vi "Main.vi"() -> ()   [LabVIEW 2019]
doc: "The myRIO Project template acquires acceleration data from the onboard accelerometer and displays the changes of acceleration values in a waveform chart."
uses:
  <vilib>/myRIO/Instrument Drivers/Onboard IO/DIO/typedefs/DIO Reference.ctl
  <vilib>/myRIO/Common/Instrument Driver Framework/Utilities/typedefs/myRIO Generic Hardware Reference.ctl
  <vilib>/myRIO/Common/Instrument Driver Framework/Utilities/typedefs/Hardware Version Enum.ctl
  <vilib>/myRIO/Common/Instrument Driver Framework/Utilities/typedefs/myRIO v1.0 Reference.ctl
  <vilib>/myRIO/Common/Instrument Driver Framework/Utilities/typedefs/Generic FPGA Reference.ctl
  <vilib>/myRIO/Common/Instrument Driver Framework/myRIO v1.0/DIO/typedefs/DIO Channels List.ctl
  <vilib>/myRIO/Common/Instrument Driver Framework/myRIO v1.0/DIO/typedefs/DIO Channels Enum.ctl
  <vilib>/userDefined/High Color/nirio_resource_hc.ctl
  <vilib>/myRIO/Instrument Drivers/Onboard IO/AI/typedefs/AI Reference.ctl
  <vilib>/myRIO/Common/Instrument Driver Framework/myRIO v1.0/AI/typedefs/AI Channels List.ctl
  <vilib>/myRIO/Common/Instrument Driver Framework/myRIO v1.0/AI/typedefs/AI Channels Enum.ctl
  <vilib>/myRIO/Common/Instrument Driver Framework/Utilities/typedefs/Analog Scaling Constants List.ctl
  <vilib>/myRIO/Common/Instrument Driver Framework/Utilities/typedefs/Analog Scaling Constants.ctl
  <vilib>/myRIO/Common/Instrument Driver Framework/Utilities/vis/Is FPGA Ref Available.vi
  <vilib>/myRIO/Common/Instrument Driver Framework/myRIO v1.0/DIO/vis/myRIO v1.1 Open DIO.vi
  <vilib>/myRIO/Instrument Drivers/Onboard IO/DIO/vis/Write.vi
  <vilib>/myRIO/Instrument Drivers/Onboard IO/DIO/vis/Read.vi
  <vilib>/myRIO/Common/Instrument Driver Framework/myRIO v1.0/AI/vis/myRIO v1.1 Open AI.vi
  <vilib>/myRIO/Instrument Drivers/Onboard IO/AI/vis/Read.vi
  <vilib>/myRIO/Common/Instrument Driver Framework/Utilities/vis/Validate Channels.vi
  <vilib>/myRIO/Common/Instrument Driver Framework/myRIO v1.0/DIO/vis/myRIO v1.0 Reserve DIO.vi
  <vilib>/myRIO/Common/Instrument Driver Framework/myRIO v1.0/AI/vis/myRIO v1.0 Reserve AI.vi
  <vilib>/myRIO/Common/Instrument Driver Framework/myRIO v1.0/UART/vis/myRIO v1.0 Close UART.vi
  <vilib>/myRIO/Common/Instrument Driver Framework/myRIO v1.0/Resource Manager/vis/myRIO v1.0 Reserve Channel List.vi
  <vilib>/myRIO/Common/Instrument Driver Framework/myRIO v1.0/DIO/vis/myRIO v1.0 Build MUX Configuration DIO.vi
  <vilib>/myRIO/Common/Instrument Driver Framework/myRIO v1.0/AI/vis/myRIO v1.0 Build MUX Configuration AI.vi
  <vilib>/myRIO/Common/Instrument Driver Framework/myRIO v1.0/Resource Manager/vis/myRIO v1.0 Reserve Channel.vi
  <vilib>/myRIO/Common/Instrument Driver Framework/myRIO v1.0/Resource Manager/vis/myRIO v1.0 Unreserve Channel.vi
  <vilib>/myRIO/Common/Instrument Driver Framework/myRIO v1.0/Resource Manager/vis/myRIO v1.0 Create Configuration List.vi
  <vilib>/myRIO/Common/Instrument Driver Framework/myRIO v1.0/Resource Manager/vis/myRIO v1.0 Build Mutex Name.vi
  <vilib>/Utility/VariantDataType/GetNumericInfo.vi
  <vilib>/Utility/error.llb/Error Cluster From Error Code.vi
  <vilib>/myRIO/Common/Instrument Driver Framework/myRIO v1.0/myRIO v1.1 Open.vi
  <vilib>/myRIO/Common/Instrument Driver Framework/Utilities/vis/IO Manager.vi
  <vilib>/myRIO/Common/Instrument Driver Framework/Utilities/vis/Configuration Manager.vi
  <vilib>/myRIO/Common/Instrument Driver Framework/myRIO v1.0/Resource Manager/vis/myRIO v1.0 Configure IO.vi
  <vilib>/myRIO/Common/Instrument Driver Framework/myRIO v1.0/myRIO v1.0 Close.vi
  <vilib>/myRIO/Common/Instrument Driver Framework/myRIO v1.0/DIO/vis/myRIO v1.0 Write DIO.vi
  <vilib>/myRIO/Common/Instrument Driver Framework/myRIO v1.0/DIO/vis/myRIO v1.0 Read DIO.vi
  <vilib>/myRIO/Common/Instrument Driver Framework/myRIO v1.0/AI/vis/myRIO v1.0 Get Scaling Constants AI.vi
  <vilib>/myRIO/Common/Instrument Driver Framework/myRIO v1.0/AI/vis/myRIO v1.0 Read AI.vi
  <vilib>/myRIO/Common/Instrument Driver Framework/Utilities/vis/FPGA Ref Manager.vi
  <vilib>/myRIO/Common/Instrument Driver Framework/myRIO v1.0/myRIO v1.0 Reset FPGA.vi
  <vilib>/myRIO/Common/Instrument Driver Framework/myRIO v1.0/IRQ/vis/myRIO v1.0 IRQ Info FGV.vi
  <vilib>/myRIO/Common/Instrument Driver Framework/myRIO v1.0/IRQ/vis/myRIO v1.0 Timer IRQ Info FGV.vi
  <vilib>/myRIO/Common/Instrument Driver Framework/myRIO v1.0/IRQ/vis/myRIO v1.0 ISR Agent.vi
  <vilib>/myRIO/Instrument Drivers/Utilities/vis/Reset Index.vi
  <vilib>/myRIO/Common/Instrument Driver Framework/myRIO v1.0/Resource Manager/vis/myRIO v1.0 Block Write Resource Manager.vi
  <vilib>/myRIO/Express VI/Onboard IO/DO/DO Express VI.xnode
  <vilib>/myRIO/Instrument Drivers/Onboard IO/DIO/vis/myRIO DIO Open.xnode
  <vilib>/myRIO/Express VI/Onboard IO/DI/DI Express VI.xnode
  <vilib>/myRIO/Express VI/Onboard IO/AI/AI Express VI.xnode
  <vilib>/myRIO/Instrument Drivers/Onboard IO/AI/vis/myRIO AI Open.xnode
  <vilib>/myRIO/Instrument Drivers/Onboard IO/DIO/DIO.lvlib
  <vilib>/myRIO/Instrument Drivers/Onboard IO/AI/AI.lvlib
  <vilib>/myRIO/Instrument Drivers/Utilities/Utilities.lvlib
panel:
  out "Array - String":string[](array[string])
  out "Numeric":dbl
  in  "Go":bool
  in  "Single/Continuous":bool
  out "INPOS":bool
  in  "Home":bool
  in  "OFF/ON":bool
  in  "L/R":bool
  out "Index":i8=-1
  in  "Displacement (cm)":u8(slide) step=2 scale=0.0..10.0
  in  "Acceleration (m/s^2)":u8(slide)=1 min=1 max=5 step=1 scale=1.0..5.0
  out "Encoder Output (V)":dbl(graph)
  out "error out":errorcluster
  in  "Stop":bool
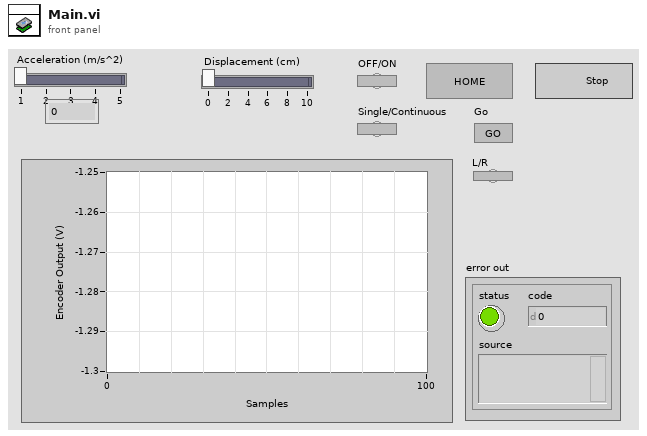
[diagram p1: front panel]
types:
  T1 = typedef "DIO.lvlib/DIO Reference.ctl" = cluster{"myRIO Reference":T2, "DIO Channels List":T6}
  T2 = typedef "myRIO Generic Hardware Reference.ctl" = cluster{"myRIO Model":T3, "myRIO Hardware Reference":T4}
  T3 = typedef "Hardware Version Enum.ctl" = enum16{"Unknown", "myRIO-1900", "myRIO-1950", "roboRIO", "NI ELVIS RIO CM", "ELVIS III"}
  T4 = typedef "myRIO v1.0 Reference.ctl" = cluster{"Generic FPGA Reference":T5, "Allow multiple opens":bool}
  T5 = typedef "Generic FPGA Reference.ctl" = refnum<k20>
  T6 = typedef "DIO Channels List.ctl" = T7[]
  T7 = typedef "DIO Channels Enum.ctl" = enum16{"Not Connected", "C/DIO0", "C/DIO1", "C/DIO2", "C/DIO3", "C/DIO4", "C/DIO5", "C/DIO6", "C/DIO7", "A/DIO0", "A/DIO1", "A/DIO2", "A/DIO3", "A/DIO4", "A/DIO5", "A/DIO6", "A/DIO7", "A/DIO8", "A/DIO9", "A/DIO10", "A/DIO11", "A/DIO12", "A/DIO13", "A/DIO14", "A/DIO15", "A/DIO16", "A/DIO17", "A/DIO18", "A/DIO19", "B/DIO0", "B/DIO1", "B/DIO2", "B/DIO3", "B/DIO4", "B/DIO5", "B/DIO6", "B/DIO7", "B/DIO8", "B/DIO9", "B/DIO10", "B/DIO11", "B/DIO12", "B/DIO13", "B/DIO14", "B/DIO15", "B/DIO16", "B/DIO17", "B/DIO18", "B/DIO19", "LED0", "LED1", "LED2", "LED3", "Button0", "DIO/DIO0", "DIO/DIO1", "DIO/DIO2", "DIO/DIO3", "DIO/DIO4", "DIO/DIO5", "DIO/DIO6", "DIO/DIO7", "DIO/DIO8", "DIO/DIO9", "SPI/CS0", "SPI/CS1", "SPI/CS2", "SPI/CS3", "LED RADIO (Green)", "LED RADIO (Red)", "LED COMM (Green)", "LED COMM (Red)", "LED MODE (Green)", "LED MODE (Red)"}
  T8 = typedef "nirio_resource_hc.ctl" = tag
  T9 = typedef "AI.lvlib/AI Reference.ctl" = cluster{"myRIO Reference":T2, "AI Channels List":T10, "AI Scaling Constants List":T12}
  T10 = typedef "AI Channels List.ctl" = T11[]
  T11 = typedef "AI Channels Enum.ctl" = enum16{"Not Connected", "AudioIn/Left", "AudioIn/Right", "C/AI0", "C/AI1", "A/AI0", "A/AI1", "A/AI2", "A/AI3", "A/AI4", "A/AI5", "A/AI6", "A/AI7", "B/AI0", "B/AI1", "B/AI2", "B/AI3", "B/AI4", "B/AI5", "B/AI6", "B/AI7", "AI/AI0", "AI/AI1", "AI/AI2", "AI/AI3", "A/AI0 (DIFF)", "A/AI1 (DIFF)", "A/AI2 (DIFF)", "A/AI3 (DIFF)", "B/AI0 (DIFF)", "B/AI1 (DIFF)", "B/AI2 (DIFF)", "B/AI3 (DIFF)"}
  T12 = typedef "Analog Scaling Constants List.ctl" = T13[]
  T13 = typedef "Analog Scaling Constants.ctl" = cluster{"LSB Weight (Volts)":dbl, "Offset (Volts)":dbl, "Signed?":bool}
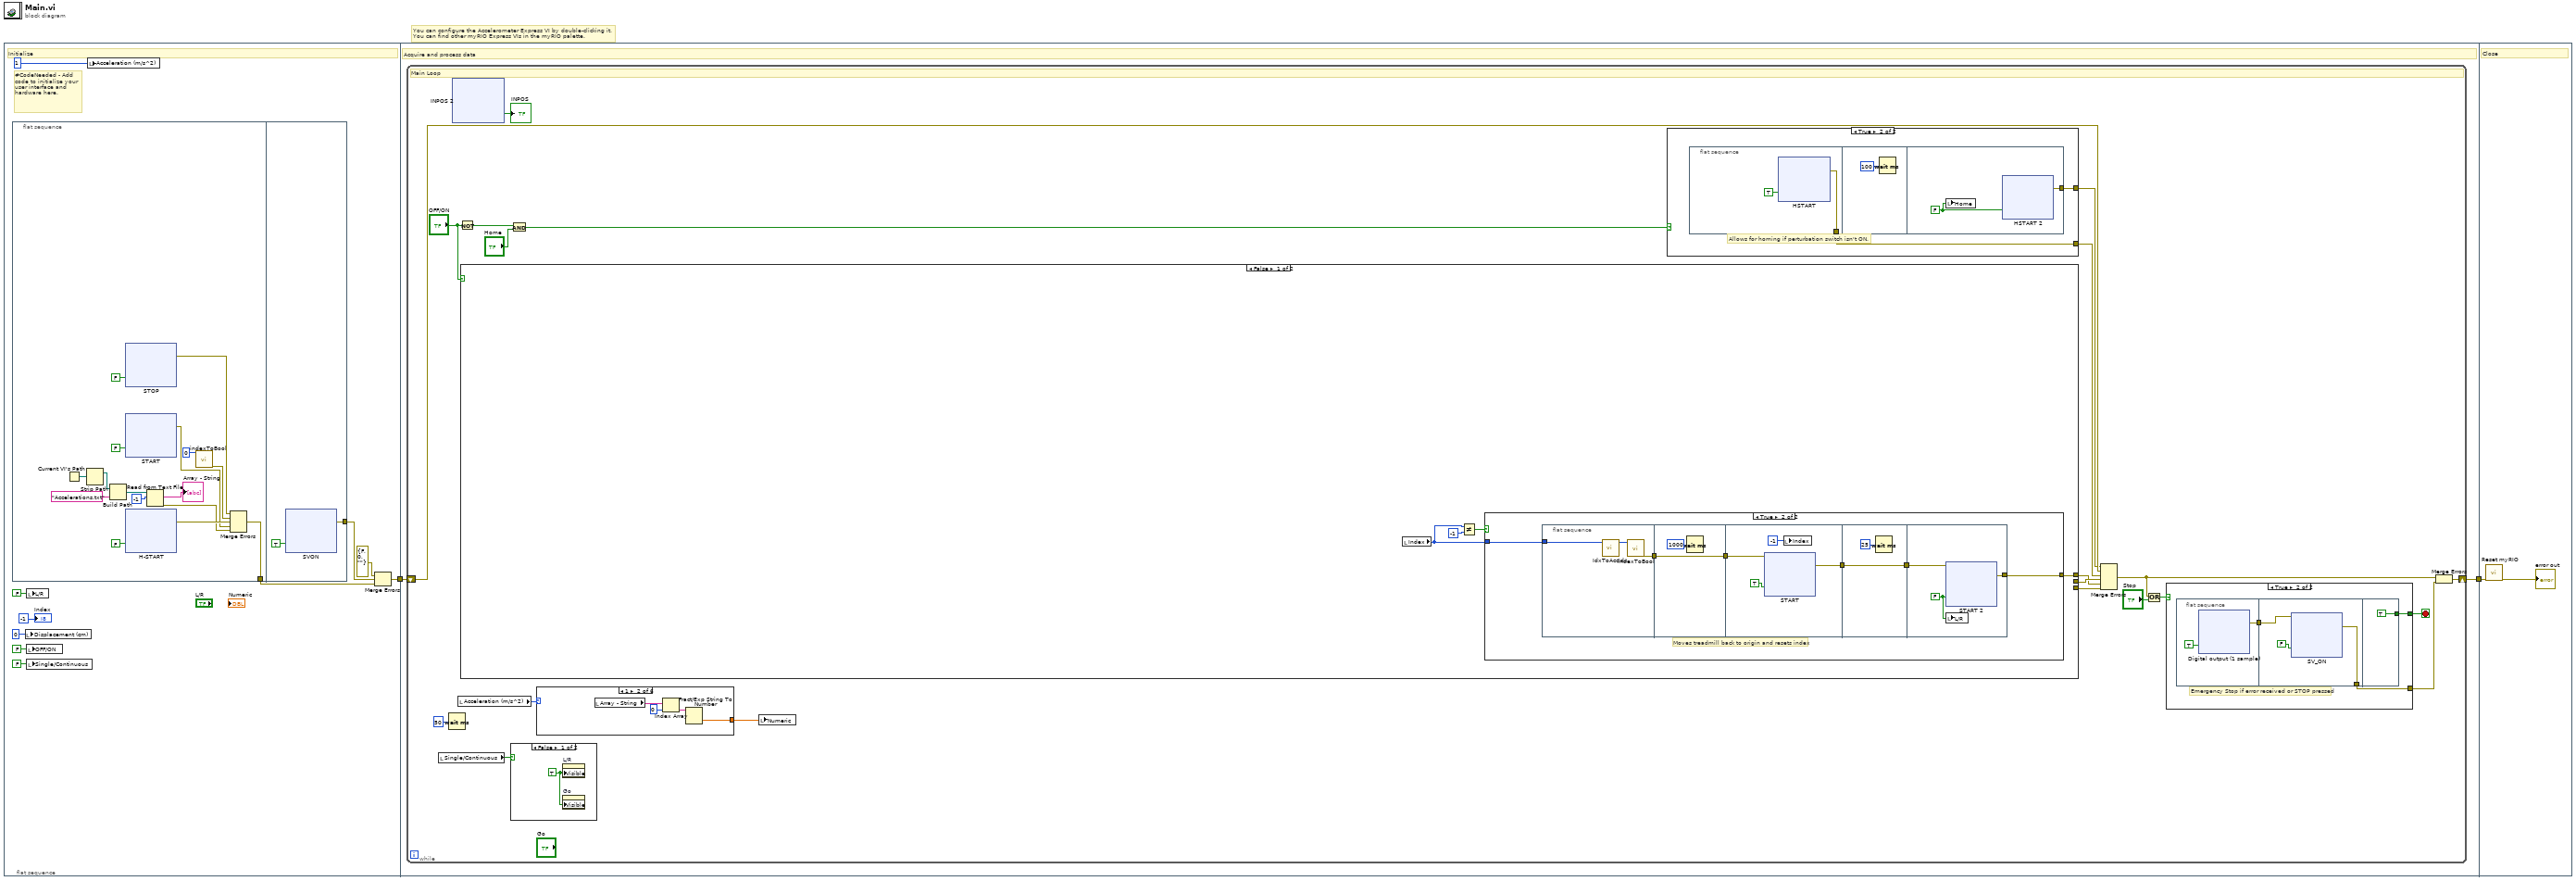
[diagram p0: block diagram]
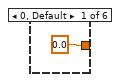
[diagram p2: hidden frame]
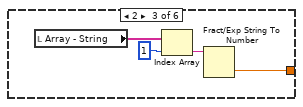
[diagram p3: hidden frame]
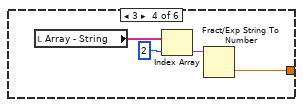
[diagram p4: hidden frame]
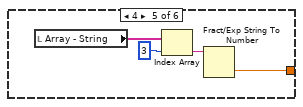
[diagram p5: hidden frame]
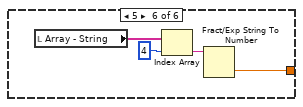
[diagram p6: hidden frame]
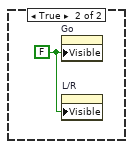
[diagram p7: hidden frame]
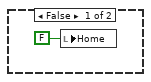
[diagram p9: hidden frame]
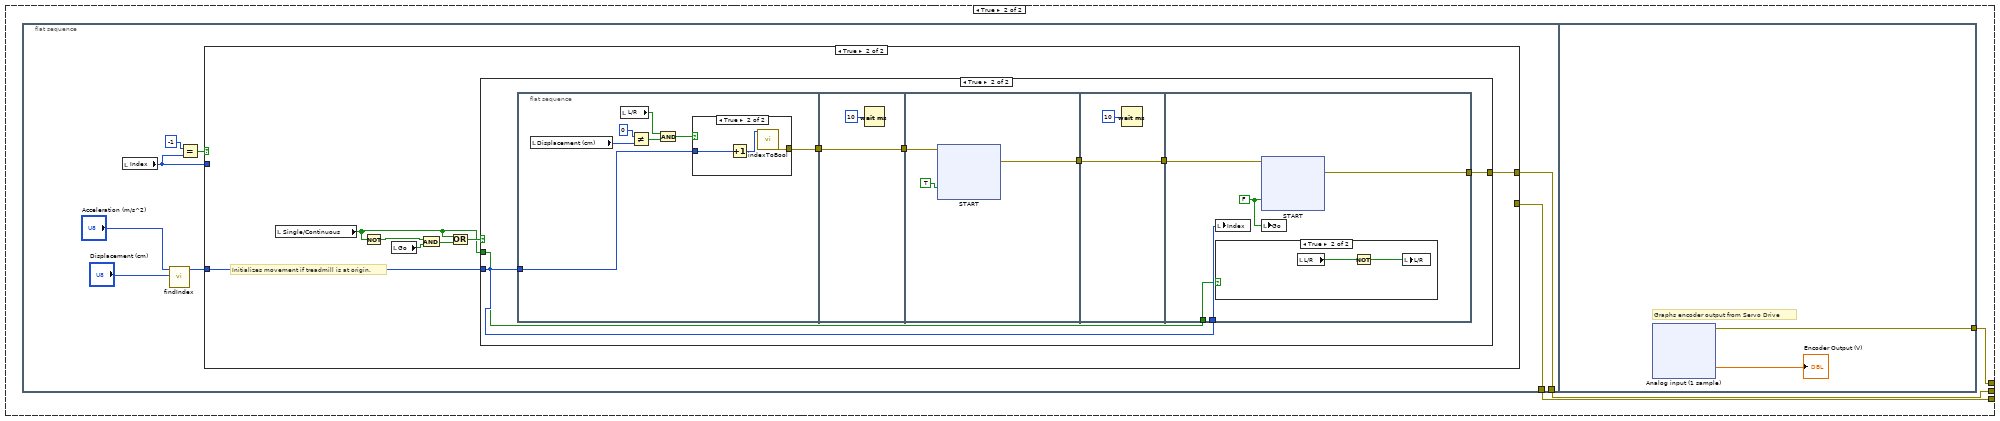
[diagram p11: hidden frame]
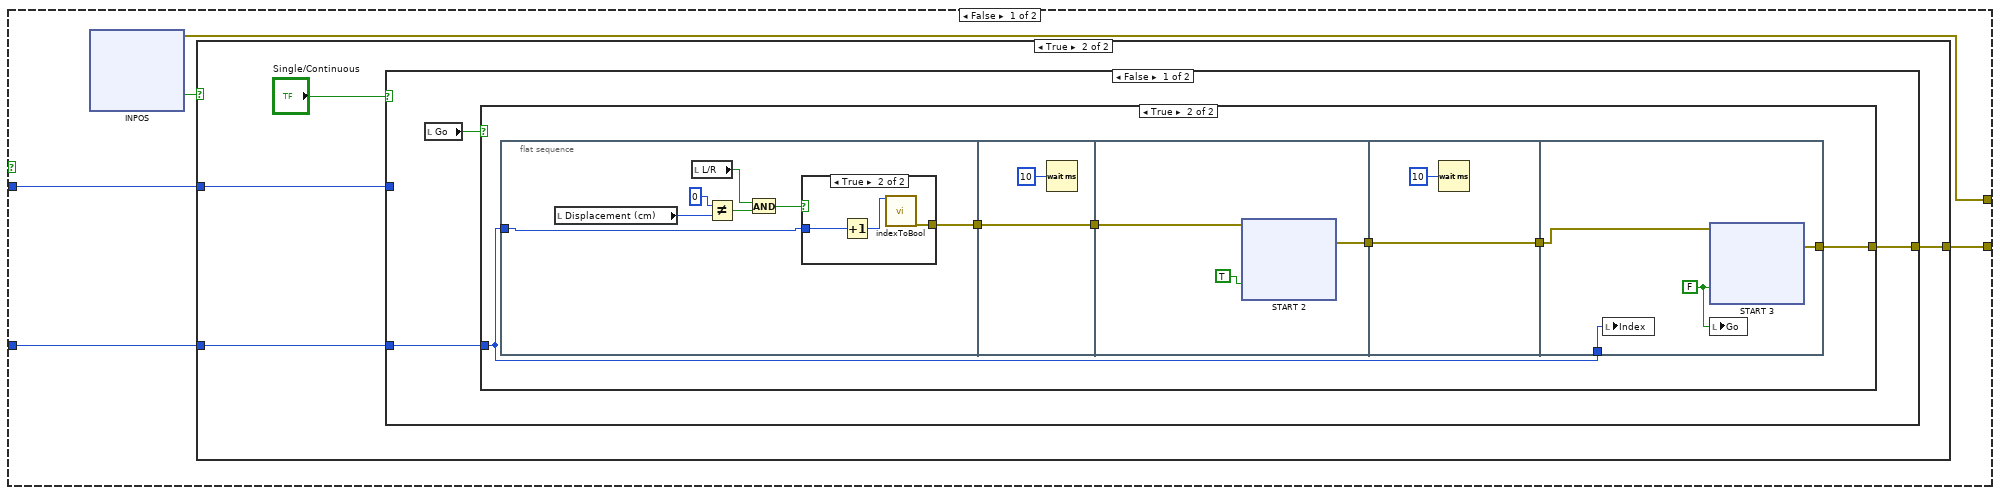
[diagram p12: hidden frame]
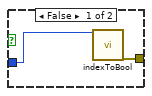
[diagram p15: hidden frame]
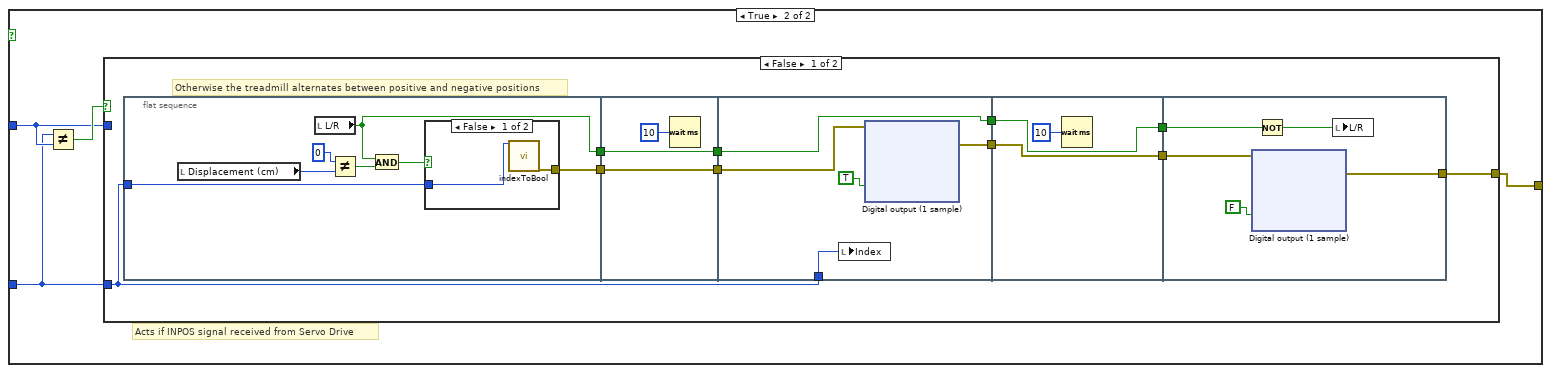
[diagram p16: hidden frame]
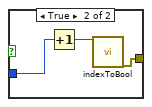
[diagram p17: hidden frame]
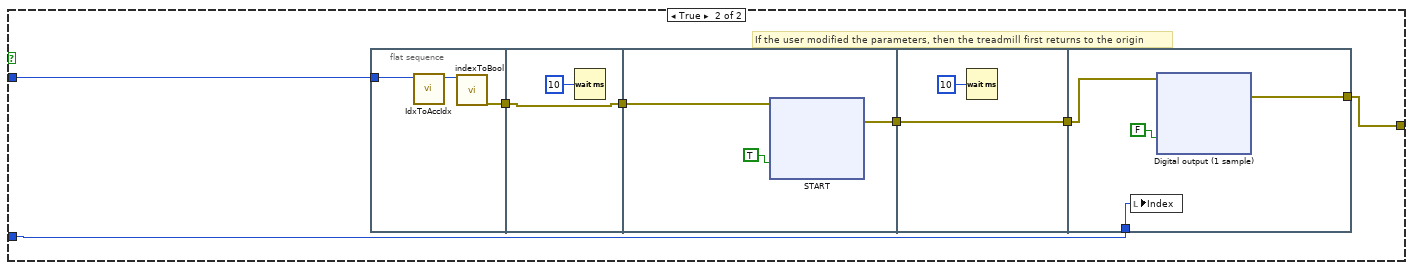
[diagram p18: hidden frame]
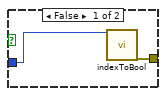
[diagram p20: hidden frame]
diagram:
  # "You can configure the Accelerometer Express VI by double-clicking it.\nYou can find other myRIO Express VIs in the myRIO palette."
  n1 = flat-sequence {
    tunnel: [w5] -> w2
    tunnel: w2 -> [w172]
    tunnel: [w171] -> w1
    tunnel: w1 -> [w1012]
    frame #0 {
      # "#CodeNeeded - Add code to initialize your user interface and hardware here."
      # "Initialize"
      n2 = flat-sequence {
        tunnel: [w24] -> w7
        tunnel: [w135] -> w6
        frame #0 {
          n3 = Current VI's Path() -> (path=w15:path)
          n4 = Strip Path(path=w15) -> (stripped path=w14:path)  [unwired: 1 out]
          n5 = Build Path(base path=w14, name or relative path="Accelerations.txt") -> (appended path=w17:path)
          n6 = xnode "STOP"("A/DIO0 (Pin 11)"=FALSE) -> ("error out"=w23:errorcluster)  [unwired: 1 in]
          n7 = xnode "START"("C/DIO2 (DIO2)"=FALSE) -> ("error out"=w25:errorcluster)  [unwired: 1 in]
          n8 = xnode "H-START"("C/DIO3 (DIO3)"=FALSE) -> ("error out"=w26:errorcluster)  [unwired: 1 in]
          n9 = Read from Text File(file (use dialog)=w17, count=-1) -> (text=→"Array - String":string[], error out=w13:errorcluster)  [unwired: 2 in, 2 out]
          n10 = call "indexToBool.vi"("Index"=0) -> ("error out"=w27:errorcluster)  [unwired: 18 in]
          n11 = Merge Errors(w23, w27, w26, w25, w13) -> (w24:errorcluster)
        }
        frame #1 {
          n12 = xnode "SVON"("C/DIO1 (DIO1)"=TRUE) -> ("error out"=w135:errorcluster)  [unwired: 1 in]
        }
      }
      n13 = local write "Displacement (cm)"(0) -> ()
      n14 = local write "L/R"(FALSE) -> ()
      n15 = local write "OFF/ON"(FALSE) -> ()
      n16 = local write "Single/Continuous"(FALSE) -> ()
      n17 = local write "Acceleration (m/s^2)"(1) -> ()
      n18 = Merge Errors(errorcluster {"status"=FALSE, "code"=0, "source"=""} ("error in (no error)"), w6, w7) -> (w5:errorcluster)
      "Index" <- -1
    }
    frame #1 {
      # "Acquire and process data"
      n19 = while {
        shift-right: [w179] -> w171
        shift-left: w172 -> [w188]
        stop <- w182 stop-if-true
        # "Main Loop"
        n20 = local read "Single/Continuous"() -> (w175:bool)
        n21 = Wait (ms)(milliseconds to wait=u32 50) -> ()  [unwired: 1 out]
        n22 = xnode "INPOS 2"() -> ("C/DIO0 (DIO0)"=→"INPOS":bool)  [unwired: 1 in, 1 out]
        n23 = local read "Acceleration (m/s^2)"() -> (w173:u8)
        n24 = Not(x="OFF/ON") -> (.not. x?=w190:bool)
        n25 = case shown="False" "OFF/ON" {
          tunnel: [_ w505] -> w186
          tunnel: [w409 w504] -> w184
          tunnel: [_ w503] -> w177
          frame False {
            n26 = local read "Index"() -> (w410:i8)
            n27 = Not Equal?(x=w410, y=-1) -> (x != y?=w411:bool)
            n28 = case shown="True" w411 {
              tunnel: w410 -> [_ w418]
              tunnel: [_ w417] -> w409
              frame False {
              }
              frame True {
                # "Moves treadmill back to origin and resets index"
                n29 = flat-sequence {
                  tunnel: w418 -> [w420]
                  tunnel: [w419] -> w414
                  tunnel: w414 -> [w423]
                  tunnel: [w423] -> w413
                  tunnel: w413 -> [w426]
                  tunnel: [w425] -> w416
                  tunnel: w416 -> [w464]
                  tunnel: [w464] -> w415
                  tunnel: [w467] -> w417
                  tunnel: w415 -> [w466]
                  frame #0 {
                    n30 = call "IdxToAccIdx.vi"("Idx"=w420) -> ("Acc. Idx"=w421:u8)  [unwired: 9 in]
                    n31 = call "indexToBool.vi"("Index"=w421) -> ("error out"=w419:errorcluster)  [unwired: 18 in]
                  }
                  frame #1 {
                    n32 = Wait (ms)(milliseconds to wait=1000) -> ()  [unwired: 1 out]
                  }
                  frame #2 {
                    n33 = xnode "START"("C/DIO2 (DIO2)"=TRUE, "error in (no error)"=w426) -> ("error out"=w425:errorcluster)
                    n34 = local write "Index"(-1) -> ()
                  }
                  frame #3 {
                    n35 = Wait (ms)(milliseconds to wait=25) -> ()  [unwired: 1 out]
                  }
                  frame #4 {
                    w465 = FALSE
                    n36 = xnode "START 2"("C/DIO2 (DIO2)"=w465, "error in (no error)"=w466) -> ("error out"=w467:errorcluster)
                    n37 = local write "L/R"(w465) -> ()
                  }
                }
              }
            }
          }
          frame True {
            n38 = flat-sequence {
              tunnel: [w508] -> w505
              tunnel: [w506] -> w503
              tunnel: [w973] -> w504
              frame #0 {
                n39 = local read "Index"() -> (w509:i8)
                n40 = call "findIndex.vi"("Disp."="Displacement (cm)", "Acc."="Acceleration (m/s^2)") -> ("Index"=w511:u8)  [unwired: 9 in]
                n41 = Equal?(x=-1, y=w509) -> (x = y?=w512:bool)
                n42 = case shown="True" w512 {
                  tunnel: w511 -> [w518 w869]
                  tunnel: w509 -> [w517 _]
                  tunnel: [w516 w868] -> w508
                  tunnel: [w515 _] -> w506
                  frame False {
                    n43 = xnode "INPOS"() -> ("C/DIO0 (DIO0)"=w514:bool, "error out"=w516:errorcluster)  [unwired: 1 in]
                    n44 = case shown="True" w514 {
                      tunnel: w518 -> [_ w556]
                      tunnel: w517 -> [_ w557]
                      tunnel: [_ w555] -> w515
                      frame False {
                      }
                      frame True {
                        n45 = case shown="False" "Single/Continuous" {
                          tunnel: w557 -> [_ w662]
                          tunnel: w556 -> [w560 w661]
                          tunnel: [w559 w660] -> w555
                          frame False {
                            n46 = local read "Go"() -> (w558:bool)
                            n47 = case shown="True" w558 {
                              tunnel: w560 -> [_ w562]
                              tunnel: [_ w561] -> w559
                              frame False {
                              }
                              frame True {
                                n48 = flat-sequence {
                                tunnel: w562 -> [w573]
                                tunnel: [w572] -> w566
                                tunnel: w566 -> [w580]
                                tunnel: [w580] -> w565
                                tunnel: w565 -> [w582]
                                tunnel: [w581] -> w564
                                tunnel: w564 -> [w620]
                                tunnel: [w620] -> w563
                                tunnel: w563 -> [w624]
                                tunnel: w562 -> [w623]
                                tunnel: [w622] -> w561
                                frame #0 {
                                n49 = local read "Displacement (cm)"() -> (w568:u8)
                                n50 = local read "L/R"() -> (w571:bool)
                                n51 = Not Equal?(x=0, y=w568) -> (x != y?=w569:bool)
                                n52 = And(x=w571, y=w569) -> (x .and. y?=w570:bool)
                                n53 = case shown="True" w570 {
                                tunnel: w573 -> [w574 w577]
                                tunnel: [w575 w578] -> w572
                                frame False {
                                n54 = call "indexToBool.vi"("Index"=w574) -> ("error out"=w575:errorcluster)  [unwired: 18 in]
                                }
                                frame True {
                                n55 = Increment(x=w577) -> (x+1=w576:u8)
                                n56 = call "indexToBool.vi"("Index"=w576) -> ("error out"=w578:errorcluster)  [unwired: 18 in]
                                }
                                }
                                }
                                frame #1 {
                                n57 = Wait (ms)(milliseconds to wait=10) -> ()  [unwired: 1 out]
                                }
                                frame #2 {
                                n58 = xnode "START 2"("C/DIO2 (DIO2)"=TRUE, "error in (no error)"=w582) -> ("error out"=w581:errorcluster)
                                }
                                frame #3 {
                                n59 = Wait (ms)(milliseconds to wait=10) -> ()  [unwired: 1 out]
                                }
                                frame #4 {
                                w621 = FALSE
                                n60 = local write "Index"(w623) -> ()
                                n61 = xnode "START 3"("C/DIO2 (DIO2)"=w621, "error in (no error)"=w624) -> ("error out"=w622:errorcluster)
                                n62 = local write "Go"(w621) -> ()
                                }
                                }
                              }
                            }
                          }
                          frame True {
                            # "Acts if INPOS signal received from Servo Drive"
                            n63 = Not Equal?(x=w661, y=w662) -> (x != y?=w663:bool)
                            n64 = case shown="False" w663 {
                              tunnel: w662 -> [_ w777]
                              tunnel: w661 -> [w673 w778]
                              tunnel: [w672 w776] -> w660
                              frame False {
                                # "Otherwise the treadmill alternates between positive and negative positions"
                                n65 = flat-sequence {
                                tunnel: [w677] -> w667
                                tunnel: w673 -> [w680]
                                tunnel: [w679] -> w665
                                tunnel: w667 -> [w688]
                                tunnel: [w688] -> w666
                                tunnel: w665 -> [w687]
                                tunnel: [w687] -> w664
                                tunnel: w673 -> [w693]
                                tunnel: [w692] -> w671
                                tunnel: w666 -> [w692]
                                tunnel: w664 -> [w690]
                                tunnel: [w689] -> w669
                                tunnel: w671 -> [w731]
                                tunnel: [w731] -> w670
                                tunnel: w669 -> [w730]
                                tunnel: [w730] -> w668
                                tunnel: w670 -> [w736]
                                tunnel: [w733] -> w672
                                tunnel: w668 -> [w732]
                                frame #0 {
                                n66 = local read "Displacement (cm)"() -> (w676:u8)
                                n67 = local read "L/R"() -> (w677:bool)
                                n68 = Not Equal?(x=0, y=w676) -> (x != y?=w674:bool)
                                n69 = And(x=w677, y=w674) -> (x .and. y?=w678:bool)
                                n70 = case shown="False" w678 {
                                tunnel: w680 -> [w681 w684]
                                tunnel: [w682 w685] -> w679
                                frame False {
                                n71 = call "indexToBool.vi"("Index"=w681) -> ("error out"=w682:errorcluster)  [unwired: 18 in]
                                }
                                frame True {
                                n72 = Increment(x=w684) -> (x+1=w683:u8)
                                n73 = call "indexToBool.vi"("Index"=w683) -> ("error out"=w685:errorcluster)  [unwired: 18 in]
                                }
                                }
                                }
                                frame #1 {
                                n74 = Wait (ms)(milliseconds to wait=10) -> ()  [unwired: 1 out]
                                }
                                frame #2 {
                                n75 = local write "Index"(w693) -> ()
                                n76 = xnode "Digital output (1 sample)"("C/DIO2 (DIO2)"=TRUE, "error in (no error)"=w690) -> ("error out"=w689:errorcluster)
                                }
                                frame #3 {
                                n77 = Wait (ms)(milliseconds to wait=10) -> ()  [unwired: 1 out]
                                }
                                frame #4 {
                                n78 = xnode "Digital output (1 sample)"("C/DIO2 (DIO2)"=FALSE, "error in (no error)"=w732) -> ("error out"=w733:errorcluster)
                                n79 = Not(x=w736) -> (.not. x?=w735:bool)
                                n80 = local write "L/R"(w735) -> ()
                                }
                                }
                              }
                              frame True {
                                # "If the user modified the parameters, then the treadmill first returns to the origin"
                                n81 = flat-sequence {
                                tunnel: w777 -> [w780]
                                tunnel: [w779] -> w773
                                tunnel: w773 -> [w783]
                                tunnel: [w783] -> w772
                                tunnel: w772 -> [w785]
                                tunnel: [w784] -> w774
                                tunnel: [w822] -> w775
                                tunnel: w774 -> [w822]
                                tunnel: w778 -> [w827]
                                tunnel: [w825] -> w776
                                tunnel: w775 -> [w824]
                                frame #0 {
                                n82 = call "IdxToAccIdx.vi"("Idx"=w780) -> ("Acc. Idx"=w781:u8)  [unwired: 9 in]
                                n83 = call "indexToBool.vi"("Index"=w781) -> ("error out"=w779:errorcluster)  [unwired: 18 in]
                                }
                                frame #1 {
                                n84 = Wait (ms)(milliseconds to wait=10) -> ()  [unwired: 1 out]
                                }
                                frame #2 {
                                n85 = xnode "START"("C/DIO2 (DIO2)"=TRUE, "error in (no error)"=w785) -> ("error out"=w784:errorcluster)
                                }
                                frame #3 {
                                n86 = Wait (ms)(milliseconds to wait=10) -> ()  [unwired: 1 out]
                                }
                                frame #4 {
                                n87 = local write "Index"(w827) -> ()
                                n88 = xnode "Digital output (1 sample)"("C/DIO2 (DIO2)"=FALSE, "error in (no error)"=w824) -> ("error out"=w825:errorcluster)
                                }
                                }
                              }
                            }
                          }
                        }
                      }
                    }
                  }
                  frame True {
                    # "Initializes movement if treadmill is at origin."
                    n89 = local read "Single/Continuous"() -> (w863:bool)
                    n90 = Not(x=w863) -> (.not. x?=w866:bool)
                    n91 = local read "Go"() -> (w865:bool)
                    n92 = And(x=w866, y=w865) -> (x .and. y?=w864:bool)
                    n93 = Or(x=w863, y=w864) -> (x .or. y?=w867:bool)
                    n94 = case shown="True" w867 {
                      tunnel: w869 -> [_ w872]
                      tunnel: [_ w871] -> w868
                      tunnel: w863 -> [_ w870]
                      frame False {
                      }
                      frame True {
                        n95 = flat-sequence {
                          tunnel: w872 -> [w882]
                          tunnel: [w883] -> w876
                          tunnel: w876 -> [w890]
                          tunnel: [w890] -> w875
                          tunnel: w875 -> [w892]
                          tunnel: [w891] -> w874
                          tunnel: w874 -> [w930]
                          tunnel: [w930] -> w873
                          tunnel: w872 -> [w935]
                          tunnel: [w934] -> w871
                          tunnel: w873 -> [w933]
                          tunnel: w870 -> [w931]
                          frame #0 {
                            n96 = local read "Displacement (cm)"() -> (w879:u8)
                            n97 = local read "L/R"() -> (w881:bool)
                            n98 = Not Equal?(x=0, y=w879) -> (x != y?=w878:bool)
                            n99 = And(x=w881, y=w878) -> (x .and. y?=w877:bool)
                            n100 = case shown="True" w877 {
                              tunnel: [w884 w888] -> w883
                              tunnel: w882 -> [w885 w886]
                              frame False {
                                n101 = call "indexToBool.vi"("Index"=w885) -> ("error out"=w884:errorcluster)  [unwired: 18 in]
                              }
                              frame True {
                                n102 = Increment(x=w886) -> (x+1=w887:u8)
                                n103 = call "indexToBool.vi"("Index"=w887) -> ("error out"=w888:errorcluster)  [unwired: 18 in]
                              }
                            }
                          }
                          frame #1 {
                            n104 = Wait (ms)(milliseconds to wait=10) -> ()  [unwired: 1 out]
                          }
                          frame #2 {
                            n105 = xnode "START"("C/DIO2 (DIO2)"=TRUE, "error in (no error)"=w892) -> ("error out"=w891:errorcluster)
                          }
                          frame #3 {
                            n106 = Wait (ms)(milliseconds to wait=10) -> ()  [unwired: 1 out]
                          }
                          frame #4 {
                            w932 = FALSE
                            n107 = local write "Index"(w935) -> ()
                            n108 = case shown="True" w931 {
                              frame False {
                              }
                              frame True {
                                n109 = local read "L/R"() -> (w936:bool)
                                n110 = Not(x=w936) -> (.not. x?=w937:bool)
                                n111 = local write "L/R"(w937) -> ()
                              }
                            }
                            n112 = xnode "START"("C/DIO2 (DIO2)"=w932, "error in (no error)"=w933) -> ("error out"=w934:errorcluster)
                            n113 = local write "Go"(w932) -> ()
                          }
                        }
                      }
                    }
                  }
                }
              }
              frame #1 {
                # "Graphs encoder output from Servo Drive"
                n114 = xnode "Analog input (1 sample)"() -> ("C/AI0 (AI0)"=→"Encoder Output (V)":dbl, "error out"=w973:errorcluster)  [unwired: 1 in]
              }
            }
          }
        }
        n115 = case shown="False" w175 {
          frame False {
            w215 = TRUE
            n116 = property on="L/R" class="Bool (strict)"("Visible"=w215) -> ()  [unwired: 2 in, 2 out]
            n117 = property on="Go" class="Bool (strict)"("Visible"=w215) -> ()  [unwired: 2 in, 2 out]
          }
          frame True {
            w216 = FALSE
            n118 = property on="Go" class="Bool (strict)"("Visible"=w216) -> ()  [unwired: 2 in, 2 out]
            n119 = property on="L/R" class="Bool (strict)"("Visible"=w216) -> ()  [unwired: 2 in, 2 out]
          }
        }
        n120 = And(x=w190, y="Home") -> (x .and. y?=w191:bool)
        n121 = case shown="1" w173 {
          tunnel: [0.0 w195 w200 w203 w207 w211] -> w174
          frame 0, Default {
          }
          frame 1 {
            n122 = local read "Array - String"() -> (w198:string[])
            n123 = Index Array(array=w198, index=0) -> (element=w196:string)
            n124 = Fract/Exp String To Number(string=w196) -> (number=w195:dbl)  [unwired: 3 in, 1 out]
          }
          frame 2 {
            n125 = local read "Array - String"() -> (w199:string[])
            n126 = Index Array(array=w199, index=1) -> (element=w202:string)
            n127 = Fract/Exp String To Number(string=w202) -> (number=w200:dbl)  [unwired: 3 in, 1 out]
          }
          frame 3 {
            n128 = local read "Array - String"() -> (w204:string[])
            n129 = Index Array(array=w204, index=2) -> (element=w206:string)
            n130 = Fract/Exp String To Number(string=w206) -> (number=w203:dbl)  [unwired: 3 in, 1 out]
          }
          frame 4 {
            n131 = local read "Array - String"() -> (w208:string[])
            n132 = Index Array(array=w208, index=3) -> (element=w210:string)
            n133 = Fract/Exp String To Number(string=w210) -> (number=w207:dbl)  [unwired: 3 in, 1 out]
          }
          frame 5 {
            n134 = local read "Array - String"() -> (w212:string[])
            n135 = Index Array(array=w212, index=4) -> (element=w214:string)
            n136 = Fract/Exp String To Number(string=w214) -> (number=w211:dbl)  [unwired: 3 in, 1 out]
          }
        }
        n137 = local write "Numeric"(w174) -> ()
        n138 = case shown="True" w191 {
          tunnel: [_ w333] -> w185
          tunnel: [_ w332] -> w176
          frame False {
            n139 = local write "Home"(FALSE) -> ()
          }
          frame True {
            # "Allows for homing if perturbation switch isn't ON."
            n140 = flat-sequence {
              tunnel: [w335] -> w333
              tunnel: [w373] -> w332
              frame #0 {
                n141 = xnode "HSTART"("C/DIO3 (DIO3)"=TRUE) -> ("error out"=w335:errorcluster)  [unwired: 1 in]
              }
              frame #1 {
                n142 = Wait (ms)(milliseconds to wait=100) -> ()  [unwired: 1 out]
              }
              frame #2 {
                w372 = FALSE
                n143 = local write "Home"(w372) -> ()
                n144 = xnode "HSTART 2"("C/DIO3 (DIO3)"=w372) -> ("error out"=w373:errorcluster)  [unwired: 1 in]
              }
            }
          }
        }
        n145 = Merge Errors(w176, w188, w185, w186, w184, w177) -> (w181:errorcluster)
        n146 = Or(x=w181, y="Stop") -> (x .or. y?=w183:bool)
        n147 = case shown="True" w183 {
          tunnel: [_ w253] -> w182
          tunnel: [_ w254] -> w180
          frame False {
          }
          frame True {
            # "Emergency Stop if error received or STOP pressed"
            n148 = flat-sequence {
              tunnel: [w255] -> w252
              tunnel: [w294] -> w254
              tunnel: w252 -> [w292]
              tunnel: [TRUE] -> w253
              frame #0 {
                n149 = xnode "Digital output (1 sample)"("A/DIO0 (Pin 11)"=TRUE) -> ("error out"=w255:errorcluster)  [unwired: 1 in]
              }
              frame #1 {
                n150 = xnode "SV_ON"("C/DIO1 (DIO1)"=FALSE, "error in (no error)"=w292) -> ("error out"=w294:errorcluster)
              }
              frame #2 {
              }
            }
          }
        }
        n151 = Merge Errors(w181, w180) -> (w179:errorcluster)
      }
    }
    frame #2 {
      # "Close"
      n152 = call <vilib>:"Reset myRIO.vi"("error in (no error)"=w1012) -> ("error out"=→"error out":errorcluster)  [unwired: 10 in]
    }
  }
